vi "Get_modify_set_Protocol.vi"() -> ()   [LabVIEW 2019]
uses:
  <vilib>/NI VeriStand/Custom Device API/Custom Device Item Ref.ctl
  Addon/Support Libraries/Protocols.lvlibp/TCP/TCP.lvclass
  C:/Dev/niveristand-instrument-addon-custom-device/Source/Addon/Support Libraries/Protocols.lvlibp/Protocol Parent/Protocol Parent.lvclass
  Addon/Support Libraries/Protocols.lvlibp/TCP/Data Access/Write IP Address.vi
  Scripting API/Scripting API.lvlib
  <vilib>/NI VeriStand/Custom Device API/Custom Device API.lvlib
panel:
  out "Instrument Addon Refnum Out":T1=18446744073709551615 format="%.0x"
  out "Error Out":errorcluster
  in  "IP Address":string
  in  "Error In":errorcluster
  in  "Instrument Addon Refnum In":T1=18446744073709551615 format="%.0x"
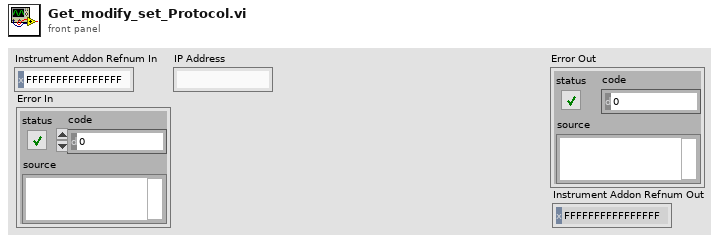
[diagram p1: front panel]
types:
  T1 = typedef "Custom Device API.lvlib/Custom Device Item Ref.ctl" = u64
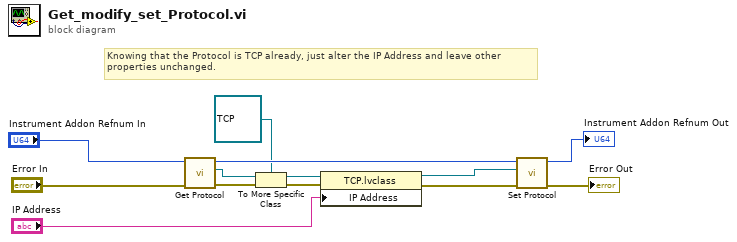
[diagram p0: block diagram]
diagram:
  # "Knowing that the Protocol is TCP already, just alter the IP Address and leave other\nproperties unchanged."
  n1 = call "Get Protocol.vi"("Error In"="Error In", "Instrument Addon Refnum In"="Instrument Addon Refnum In") -> ("Error Out"=w9:errorcluster, "Protocol"=w10:refnum<class "Protocol Parent.lvclass">, "Instrument Addon Refnum Out"=w11:T1)  [unwired: 7 in]
  n2 = To More Specific Class(target class=refnum<class "TCP.lvclass"> refnum ("Protocols.lvlibp:TCP.lvclass"), reference=w10, error in=w9) -> (specific class reference=w8:refnum<class "TCP.lvclass">, error out=w7:errorcluster)
  n3 = property class="TCP.lvclass"(reference=w8, error in=w7, "IP Address"="IP Address") -> (reference out=w3:refnum<class "TCP.lvclass">, error out=w4:errorcluster)
  n4 = call "Set Protocol.vi"("Error In"=w4, "Protocol"=w3, "Instrument Addon Refnum In"=w11) -> ("Error Out"=→"Error Out":errorcluster, "Instrument Addon Refnum Out"=→"Instrument Addon Refnum Out":T1)  [unwired: 7 in]
